vi "Filter Input Term.vi"(7 "InnerTerminal in":refnum<vi>, 11 "Wire.Terms[] in":refnum<vi>[](array[refnum])) -> (3 "Wire.Terms[] out":refnum<vi>[](array[refnum]))   [LabVIEW 2017, in "CSM-Helper.lvclass"]
uses:
  CSM-Helper.lvclass
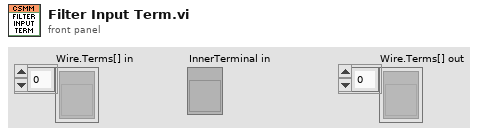
[diagram p1: front panel]
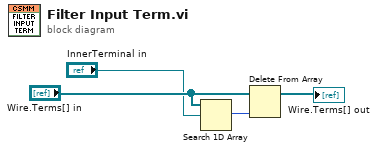
[diagram p0: block diagram]
diagram:
  n1 = Search 1D Array(1D array="Wire.Terms[] in", element="InnerTerminal in") -> (index of element=w3:i32)  [unwired: 1 in]
  n2 = Delete From Array(array="Wire.Terms[] in", index=w3) -> (array with subset deleted=→"Wire.Terms[] out":refnum<vi>[])  [unwired: 1 in, 1 out]
